vi "SS2 Live_Init Live Acquisition.vi"(8 "error in (no error)":errorcluster, 11 "SS2 Live Internal Variables in":T3={"okCFrontPanelDevices Refnum"=refnum, "Device Refnum"=refnum, "Display Image"=refnum, "# Live Images"=0, "relative s"=0.0, "# Image Sets"=0, "Message"="", "Current Image Set"=0, "# Datasets"=0, "Current Dataset"=0, "Live Mode"=FALSE, "Recording Mode"=FALSE, "Record Button"=refnum, "Live Button"=refnum, "SS2 Live Gate Data Q Name"="SS2 Live Gate Data Q", "Discard First Image"=FALSE, "Image Information"={"Save ROI Only"=FALSE, "Left"=0, "Top"=0, "Right"=0, "Bottom"=0, "Use Current ROI"=FALSE}, "Image Binning Options"={"Use Image Binning"=FALSE, "X Bin"=1, "Y Bin"=1}} {"Image Binning Options"."Y Bin" min=1; "Image Binning Options"."X Bin" min=1}) -> (0 "error out":errorcluster, 1 "Message":string, 2 "SS2 Live Atomic Action":T1={"SS2 Q Event"=enum."Idle", "Data"=variant}, 3 "SS2 Live Internal Variables out":T3={"okCFrontPanelDevices Refnum"=refnum, "Device Refnum"=refnum, "Display Image"=refnum, "# Live Images"=0, "relative s"=0.0, "# Image Sets"=0, "Message"="", "Current Image Set"=0, "# Datasets"=0, "Current Dataset"=0, "Live Mode"=FALSE, "Recording Mode"=FALSE, "Record Button"=refnum, "Live Button"=refnum, "SS2 Live Gate Data Q Name"="SS2 Live Gate Data Q", "Discard First Image"=FALSE, "Image Information"={"Save ROI Only"=FALSE, "Left"=0, "Top"=0, "Right"=0, "Bottom"=0, "Use Current ROI"=FALSE}, "Image Binning Options"={"Use Image Binning"=FALSE, "X Bin"=1, "Y Bin"=1}} {"Image Binning Options"."Y Bin" min=1; "Image Binning Options"."X Bin" min=1})   [LabVIEW 2019]
uses:
  SS2 Live Internal Variables.ctl
  C:/UCLA Thinkpad Google Drive/LabVIEW 2019 SP1/builds/SS2 Live Distribution/Opal Kelly/C# Wrapper/libFrontPanel-csharp.dll
  Opal Kelly/C# Wrapper/libFrontPanel-csharp.dll
  <vilib>/vision/Image Controls.llb/IMAQ Image.ctl
  SS2 Live_Image ROI Information.ctl
  Phasor/Image Binning Options.ctl
  SS2 Q [Element].ctl
  SS2 Q Event List.ctl
  SS2 Live_Settings List.ctl
  Variant/Variant to Data/Variant to Data.lvlib
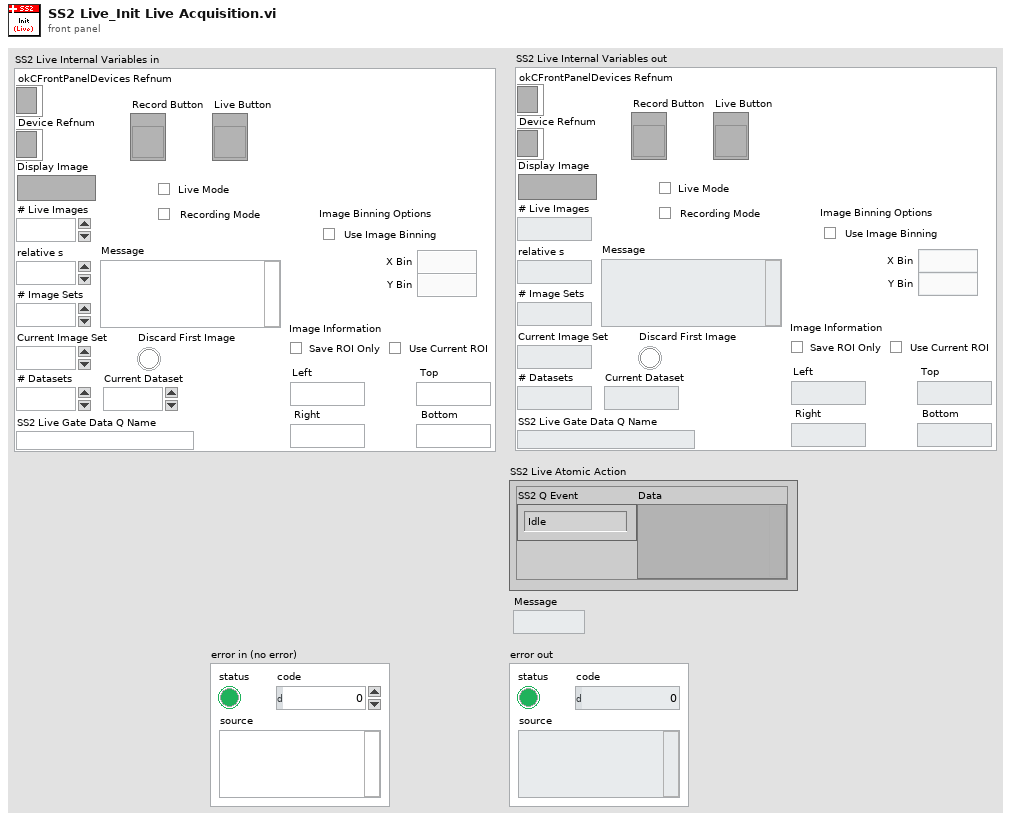
[diagram p1: front panel]
types:
  T1 = typedef "SS2 Q [Element].ctl" = cluster{"SS2 Q Event":T2, "Data":variant}
  T2 = typedef "SS2 Q Event List.ctl" = enum16{"---- UI ----", "Idle", "Initialization", "FPGA Status", "Quit", "---- DAQ ----", "Start Recording", "Start Live Acquisition", "Initialize Recording Mode", "Initialize FPGA (Live Mode)", "Get Image Set", "Get Single Image", "Update Image Display", "Stop Live Acquisition", "Stop Data Recording", "Stop Data Saving", "---- Image ----", "Copy Data to Clipboard", "Set Image Palette", "Save Displayed Image with Overlay", "Save Image Data as TIFF"}
  T3 = typedef "SS2 Live Internal Variables.ctl" = cluster{"okCFrontPanelDevices Refnum":refnum<k24>, "Device Refnum":refnum<k24>, "Display Image":T4, "# Live Images":i32, "relative s":dbl, "# Image Sets":i32, "Message":string, "Current Image Set":i32, "# Datasets":i32, "Current Dataset":i32, "Live Mode":bool, "Recording Mode":bool, "Record Button":refnum<vi>, "Live Button":refnum<vi>, "SS2 Live Gate Data Q Name":string, "Discard First Image":bool, "Image Information":T5, "Image Binning Options":T6}
  T4 = typedef "IMAQ Image.ctl" = refnum<image>
  T5 = typedef "SS2 Live_Image ROI Information.ctl" = cluster{"Save ROI Only":bool, "Left":u16, "Top":u16, "Right":u16, "Bottom":u16, "Use Current ROI":bool}
  T6 = typedef "Image Binning Options.ctl" = cluster{"Use Image Binning":bool, "X Bin":i32, "Y Bin":i32}
  T7 = typedef "SS2 Live_Settings List.ctl" = enum16{"FPGA:Bitfile Path", "FPGA:Bitfile Version", "Acquisition Parameters:SS2 DAQ Parameters", "Acquisition Parameters:Gate Configuration Array", "Acquisition Parameters:Buffer Size (# Gates)", "File Information:File Information", "File Information:# Datasets in Series", "Image Parameters:Image ROI Information", "Image Parameters:Image Binning Options", "UI Parameters:Histogram Bins Number"}
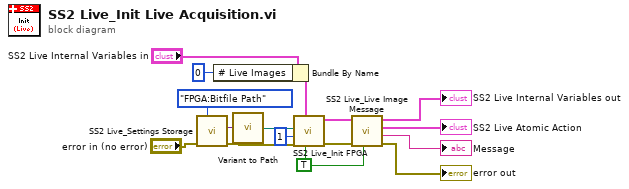
[diagram p0: block diagram]
diagram:
  w1 = TRUE ("Live Mode")
  n1 = call "SS2 Live_Settings Storage.vi"("Error In"="error in (no error)", "Settings List"=SS2_Live_Settings_List."FPGA:Bitfile Path") -> ("Error Out"=w9:errorcluster, "Variant Data out"=w11:variant)  [unwired: 8 in]
  n2 = Bundle By Name(cluster="SS2 Live Internal Variables in", "# Live Images"=0) -> (w6:T3)
  n3 = call "Variant to Path.vi"("Variant"=w11) -> ("Path"=w7:path)  [unwired: 8 in]
  n4 = call "SS2 Live_Init FPGA.vi"("Live Mode"=w1, "Error In"=w9, "Current Image Set"=1, "FPGA bitfile Path"=w7, "SS2 Live Internal Variables in"=w6) -> ("Error Out"=w5:errorcluster, "SS2 Live Internal Variables out"=w4:T3)  [unwired: 3 in, 2 out]
  n5 = call "SS2 Live_Live Image Message.vi"("Init"=w1, "error in (no error)"=w5, "SS2 Live Internal Variables"=w4) -> ("error out"=→"error out":errorcluster, "Message"=→"Message":string, "SS2 Live Atomic Action"=→"SS2 Live Atomic Action":T1, "SS2 Live Internal Variables"=→"SS2 Live Internal Variables out":T3)  [unwired: 5 in]
